vi "_range_table_coerce_int64.vi"(7 "Attribute":T1={"Identifier"="", "Descriptive Name"="", "Data Type"=enum."Integer 32", "Command"="", "Access"=enum."Read/Write", "Range Table"="", "Read Callback"="", "Write Callback"="", "Supported Models"="", "Instrument Options"="", "Index"=0, "OPC Wait"=FALSE, "No Status Check"=FALSE, "Cache Only"=FALSE}, 8 "error in":errorcluster caption="error in (no error)", 10 "Int64 in":i64, 11 "VISA resource name":refnum<visa-resource-name>) -> (0 "error out":errorcluster, 2 "Int64 out":i64, 3 "VISA resource name out":refnum<visa-resource-name>)   [LabVIEW 2020, in "Rohde&Schwarz RTx Oscilloscopes.lvlib" / "rsidr_core.lvlib"]
uses:
  rsidr_core.lvlib
  type_Attribute.ctl
  type_Attribute_Data_Type.ctl
  type_ReadWriteAccess.ctl
  _type_Operation_Fgv_RangeTable.ctl
  type_Error_Codes.ctl
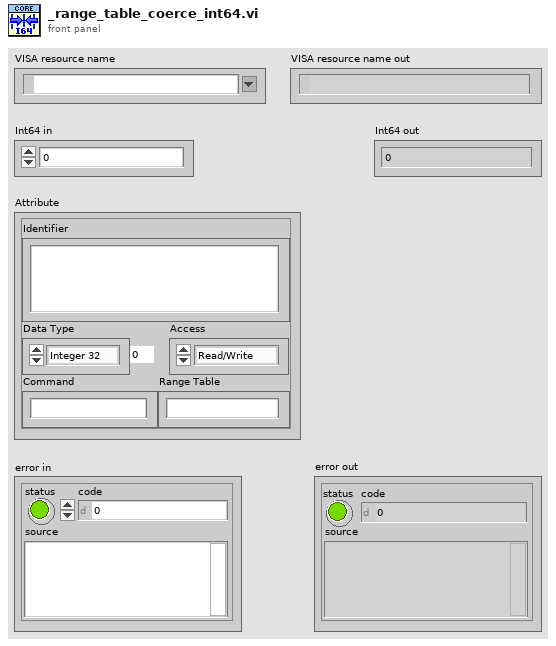
[diagram p1: front panel]
types:
  T1 = typedef "Rohde&Schwarz RTx Oscilloscopes.lvlib/rsidr_core.lvlib/type_Attribute.ctl" = cluster{"Identifier":string, "Descriptive Name":string, "Data Type":T2, "Command":string, "Access":T3, "Range Table":string, "Read Callback":string, "Write Callback":string, "Supported Models":string, "Instrument Options":string, "Index":i32, "OPC Wait":bool, "No Status Check":bool, "Cache Only":bool}
  T2 = typedef "Rohde&Schwarz RTx Oscilloscopes.lvlib/rsidr_core.lvlib/type_Attribute_Data_Type.ctl" = enum16{"Integer 32", "Double", "String", "Boolean", "None", "Integer 64", "RawString"}
  T3 = typedef "Rohde&Schwarz RTx Oscilloscopes.lvlib/rsidr_core.lvlib/type_ReadWriteAccess.ctl" = enum16{"Read Only", "Write Only", "Read/Write"}
  T4 = typedef "Rohde&Schwarz RTx Oscilloscopes.lvlib/rsidr_core.lvlib/_type_Operation_Fgv_RangeTable.ctl" = enum16{"Initialize", "Check", "Coerce", "Get Command String", "Get Numeric Value", "Get Default Value", "Get Range Table Type"}
  T5 = typedef "Rohde&Schwarz RTx Oscilloscopes.lvlib/rsidr_core.lvlib/type_Error_Codes.ctl" = enum16{"No_error", "VISA_err_ResourceNotFound", "VISA_err_Timeout", "VISA_warn_MoreDataAvailable", "RS_err_MissingCallback", "RS_err_InvalidAttribute", "RS_err_InvalidValue", "RS_err_UnknownResource", "RS_err_AlreadyInitialized", "RS_err_InstrumentStatus", "RS_err_BadRepCapName", "RS_err_TypesMismatch", "RS_err_ValueNotSupported", "RS_err_InvalidRngTable", "RS_err_IDqueryFail", "RS_err_UnexpResponse", "VISA_warn_ConfigNotLoaded", "RS_err_AttributeNotReadable", "RS_err_AttributeNotWritable", "RS_err_InstrumentType", "RS_err_InstrumentOption", "VISA_err_InvalidSize", "RS_err_ReliabilityIndicator", "VISA_warn_UnknownStatus", "VISA_warn_TermCharRead", "VISA_err_IO_error", "RS_err_FunctionNotSupported", "VISA_warn_QueueEmpty"}
  T6 = typedef "Rohde&Schwarz RTx Oscilloscopes.lvlib/rsidr_core.lvlib/_type_RangeTable_Type.ctl" = enum16{"Ranged", "Coerced", "Discrete"}
  T7 = typedef "Rohde&Schwarz RTx Oscilloscopes.lvlib/rsidr_core.lvlib/type_Session_Data.ctl" = cluster{"IDN string":string, "Instrument FW":string, "Instr type":string, "Instr type for err. msg.":string, "Installed Options":string[], "Ignore Error Messages":string, "Logging params":variant, "OPC Timeout":i32, "VISA Timeout":i32, "STB Poll VISA Timeout":i32, "Additional Flags":i32, "Wait Before Read":i32, "Wait Before Write":i32, "Option String Flags":i32, "IO Segment Size":i64, "VISA Access Mode":T8, "Interface Type":T9, "OPC Wait Mode":T10, "Bin Float Number  Format":T11, "Bin Integer Number Format":T12, "Simulate":bool, "VXIcapable":bool, "Duplicate Session":bool, "Add LF to Write":bool, "Logging":bool, "Fast Sweep":bool, "Query Instrument Status":bool, "Check Range":bool, "Check Options":bool, "OPC-sync Attr Writes":bool, "OPC-sync Attr Queries":bool}
  T8 = typedef "Rohde&Schwarz RTx Oscilloscopes.lvlib/rsidr_core.lvlib/type_VisaAccessMode.ctl" = u16
  T9 = typedef "Rohde&Schwarz RTx Oscilloscopes.lvlib/rsidr_core.lvlib/type_InterfaceType.ctl" = enum16{"Unknown", "GPIB", "VXI", "GPIB_VXI", "ASRL", "PXI", "TCPIP", "USB", "SOCKET"}
  T10 = typedef "Rohde&Schwarz RTx Oscilloscopes.lvlib/rsidr_core.lvlib/type_OPC_Wait_Mode.ctl" = enum16{"STBpolling", "STBpollingSlow", "STBpollingSuperSlow", "ServiceRequest", "OPCquery"}
  T11 = typedef "Rohde&Schwarz RTx Oscilloscopes.lvlib/rsidr_core.lvlib/type_Binary_Float_Number_Format.ctl" = enum16{"Float_4_Bytes_Swapped", "Float_4_Bytes", "Double_8_Bytes_Swapped", "Double_8_Bytes"}
  T12 = typedef "Rohde&Schwarz RTx Oscilloscopes.lvlib/rsidr_core.lvlib/type_Binary_Integer_Number_Format.ctl" = enum16{"Int32_4_Bytes_Swapped", "Int32_4 Bytes", "Int16_2_Bytes_Swapped", "Int16_2_Bytes"}
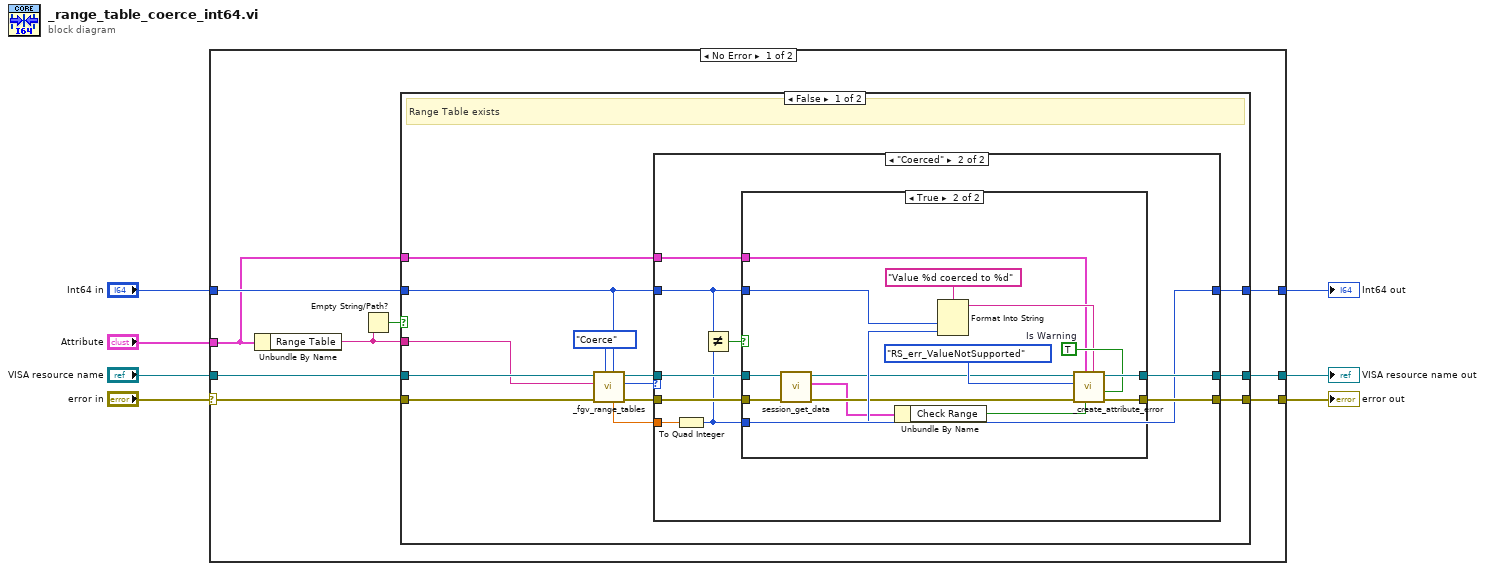
[diagram p0: block diagram]
diagram:
  n1 = case shown="No Error" "error in" {
    selector: "error in" -> [w16 w63]
    tunnel: "VISA resource name" -> [w15 w64]
    tunnel: [w10 w64] -> w2
    tunnel: [w11 w63] -> w3
    tunnel: "Attribute" -> [w8 _]
    tunnel: "Int64 in" -> [w12 w62]
    tunnel: [w9 w62] -> w1
    frame No Error {
      n2 = Unbundle By Name(w8) -> ("Range Table"=w13:string)
      n3 = Empty String/Path?(string/path=w13) -> (empty?=w14:bool)
      n4 = case shown="False" w14 {
        tunnel: w16 -> [w29 w61]
        tunnel: w15 -> [w28 w60]
        tunnel: w13 -> [w26 _]
        tunnel: w12 -> [w24 w59]
        tunnel: [w19 w61] -> w11
        tunnel: [w18 w60] -> w10
        tunnel: [w25 w59] -> w9
        tunnel: w8 -> [w17 _]
        frame False {
          # "Range Table exists"
          n5 = call "_fgv_range_tables.vi"("Numeric Value in (0.0)"=w24, "Operation"=_type_Operation_Fgv_RangeTable."Coerce", "error in"=w29, "Range Table ID in"=w26, "VISA resource name"=w28) -> ("error out"=w21:errorcluster, "Range Table Type out"=w22:T6, "VISA resource name out"=w20:refnum<visa-resource-name>, "Numeric Value out"=w23:dbl)  [unwired: 2 in, 1 out]
          n6 = case shown="\"Coerced\"" w22 {
            tunnel: w23 -> [_ w41]
            tunnel: w24 -> [w32 w35]
            tunnel: [w32 w34] -> w25
            tunnel: w20 -> [w30 w39]
            tunnel: w21 -> [w31 w40]
            tunnel: [w31 w38] -> w19
            tunnel: [w30 w37] -> w18
            tunnel: w17 -> [_ w33]
            frame "Ranged", "Discrete" {
            }
            frame "Coerced" {
              n7 = To Quad Integer(1:w41) -> (0:w34:i64)
              n8 = Not Equal?(x=w35, y=w34) -> (x != y?=w36:bool)
              n9 = case shown="True" w36 {
                tunnel: w35 -> [_ w58]
                tunnel: w40 -> [w43 w50]
                tunnel: w39 -> [w42 w49]
                tunnel: [w43 w56] -> w38
                tunnel: [w42 w55] -> w37
                tunnel: w34 -> [_ w57]
                tunnel: w33 -> [_ w51]
                frame False {
                }
                frame True {
                  w54 = TRUE  # Is Warning
                  n10 = call "session_get_data.vi"("error in"=w50, "VISA resource name"=w49) -> ("error out"=w48:errorcluster, "Session User Data out"=w46:T7, "VISA resource name out"=w47:refnum<visa-resource-name>)  [unwired: 6 in, 1 out]
                  n11 = Unbundle By Name(w46) -> ("Check Range"=w45:bool)
                  n12 = Format Into String(format string="Value %d coerced to %d" ("string"), w58, w57) -> (resulting string=w53:string)  [unwired: 2 in, 1 out]
                  n13 = call "_create_attribute_error.vi"("Is Warning (False)"=w54, "Error Elaboration (\"\")"=w53, "Error creation enabled (T)"=w45, "Attribute"=w51, "error in"=w48, "Error Enum in"=type_Error_Codes."RS_err_ValueNotSupported", "VISA resource name"=w47) -> ("error out"=w56:errorcluster, "VISA resource name out"=w55:refnum<visa-resource-name>)  [unwired: 3 in]
                }
              }
            }
          }
        }
        frame True {
          # "No Range Table"
        }
      }
    }
    frame Error {
    }
  }
  "error out" <- w3
  "VISA resource name out" <- w2
  "Int64 out" <- w1
